vi "CreateSocketHandler.vi"(5 "Name":string, 7 "Port":i32, 8 "error in (no error)":errorcluster, 10 "Address (127.0.0.1)":string="127.0.0.1", 11 "Logger in":refnum<class "Logger.lvclass">) -> (0 "error out":errorcluster, 2 "SocketHandler":refnum<class "SocketHandler.lvclass">, 3 "Logger out":refnum<class "Logger.lvclass">)   [LabVIEW 2022 SP3, in "Logger.lvlib" / "Logger.lvclass"]
uses:
  Logger.lvclass
  Logger.lvclass/Logger.ctl
  SocketHandler/SocketHandler.lvclass
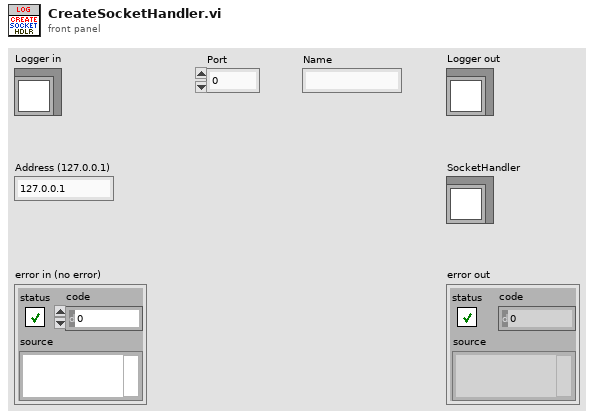
[diagram p1: front panel]
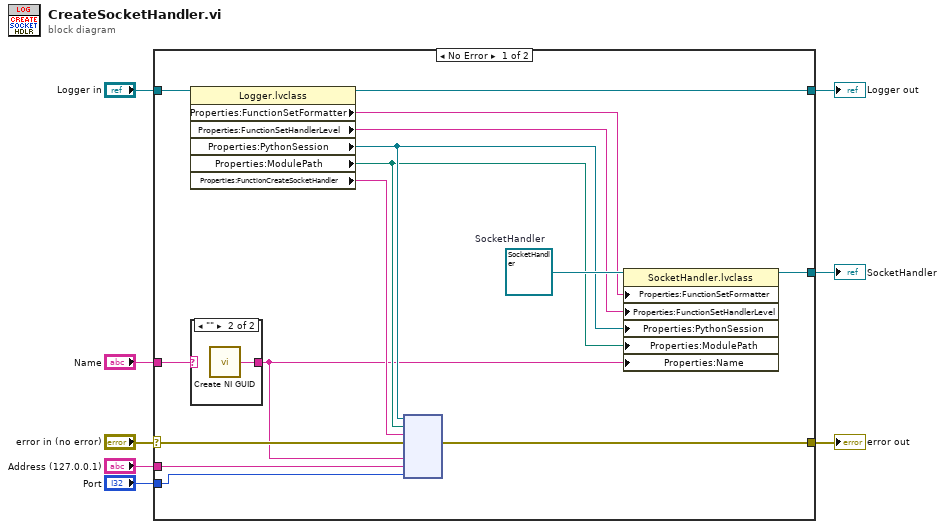
[diagram p0: block diagram]
diagram:
  n1 = case shown="No Error" "error in (no error)" {
    selector: "error in (no error)" -> [w21 w27]
    tunnel: [w19 w27] -> w5
    tunnel: [w22 w26] -> w7
    tunnel: "Logger in" -> [w23 w26]
    tunnel: "Address (127.0.0.1)" -> [w10 _]
    tunnel: "Port" -> [w11 _]
    tunnel: [w16 _] -> w4
    tunnel: "Name" -> [w17 _]
    frame No Error {
      w18 = refnum<class "SocketHandler.lvclass"> refnum  # SocketHandler
      n2 = property class="Logger.lvclass"(reference=w23) -> (reference out=w22:refnum<class "Logger.lvclass">, "Properties:FunctionSetFormatter"=w15:string, "Properties:FunctionSetHandlerLevel"=w14:string, "Properties:PythonSession"=w13:refnum<k35>, "Properties:ModulePath"=w12:path, "Properties:FunctionCreateSocketHandler"=w20:string)  [unwired: 1 in, 1 out]
      n3 = case shown="\"\"" w17 {
        selector: w17 -> [w24 _]
        tunnel: [w24 w25] -> w9
        frame Default {
        }
        frame "" {
          n4 = call <vilib>:"Create NI GUID.vi"() -> ("NI GUID"=w25:string)
        }
      }
      n5 = node(w13, w12, w20, w21, w9, w10, w11) -> (w19:errorcluster)  [unwired: 5 in, 3 out]
      n6 = property class="SocketHandler.lvclass"(reference=w18, "Properties:FunctionSetFormatter"=w15, "Properties:FunctionSetHandlerLevel"=w14, "Properties:PythonSession"=w13, "Properties:ModulePath"=w12, "Properties:Name"=w9) -> (reference out=w16:refnum<class "SocketHandler.lvclass">)  [unwired: 1 in, 1 out]
    }
    frame Error {
    }
  }
  "error out" <- w5
  "Logger out" <- w7
  "SocketHandler" <- w4
